vi "Convert_SJ_Cluster.vi"(3 "SJ Data String":string, 4 "Mode":T1(ring), 5 "SJ Data":T2={"Do (mm)"=3.0, "Dc (mm)"=0.039, "Ho (mm)"=0.01, "Hc (mm)"=0.006, "K"=1.251, "beta"=1.039, "Vc (m^3)"=0.0, "Vo (m^3)"=0.0}) -> (0 "SJ Data String Out":string, 2 "SJ Data Out":T2)   [LabVIEW 2022 SP3]
uses:
  Controls/SJ_Data_Cluster.ctl
  <vilib>/Utility/error.llb/DialogType.ctl
panel:
  out "error out":errorcluster
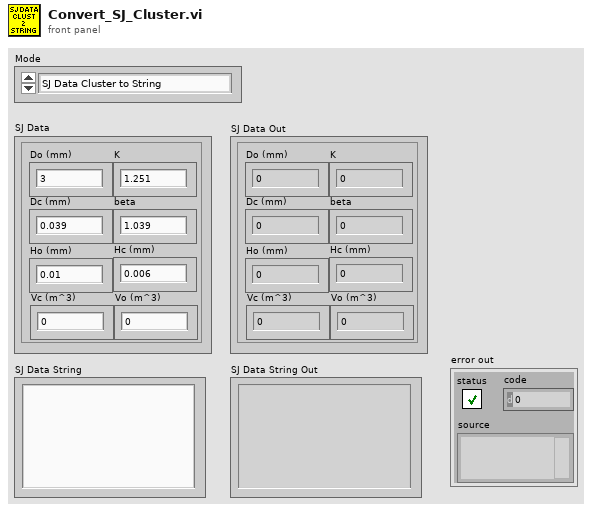
[diagram p1: front panel]
types:
  T1 = enum16{"SJ Data Cluster to String", "String to SJ Data Cluster"}
  T2 = typedef "SJ_Data_Cluster.ctl" = cluster{"Do (mm)":dbl, "Dc (mm)":dbl, "Ho (mm)":dbl, "Hc (mm)":dbl, "K":dbl, "beta":dbl, "Vc (m^3)":dbl, "Vo (m^3)":dbl}
  T3 = enum16{"big-endian, network order", "native, host order", "little-endian"}
  T4 = typedef "DialogType.ctl" = u16
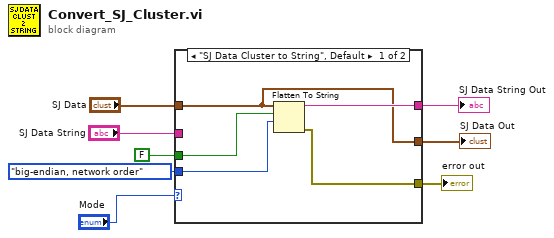
[diagram p0: block diagram]
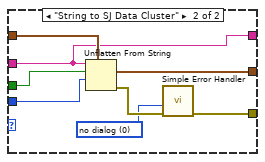
[diagram p2: hidden frame]
diagram:
  n1 = case shown="\"SJ Data Cluster to String\", Default" "Mode" {
    tunnel: "SJ Data String" -> [_ w17]
    tunnel: "SJ Data" -> [w10 w21]
    tunnel: [w10 w20] -> w2
    tunnel: FALSE ("data includes array or string size? (T)") -> [w13 w19]
    tunnel: T3."big-endian, network order" ("byte order (0:big-endian, network order)") -> [w12 w18]
    tunnel: [w11 w17] -> w3
    tunnel: [w9 w14] -> w1
    frame "SJ Data Cluster to String", Default {
      n2 = Flatten To String(anything=w10, prepend array or string size? (T)=w13, byte order (0:big-endian, network order)=w12) -> (data string=w11:string, error out=w9:errorcluster)  [unwired: 1 in, 1 out]
    }
    frame "String to SJ Data Cluster" {
      w15 = T4 0 items=["no dialog", "OK message", "continue or stop message", "OK message + warnings", "continue/stop + warnings"] ("type of dialog (OK msg:1)")
      n3 = Unflatten From String(type=w21, binary string=w17, data includes array or string size? (T)=w19, byte order (0:big-endian, network order)=w18) -> (value=w20:T2, error out=w16:errorcluster)  [unwired: 1 in, 1 out]
      n4 = call <vilib>:"Simple Error Handler.vi"("type of dialog (OK msg:1)"=w15, "error in (no error)"=w16) -> ("error out"=w14:errorcluster)  [unwired: 3 in, 4 out]
    }
  }
  "SJ Data String Out" <- w3
  "SJ Data Out" <- w2
  "error out" <- w1
